vi "_FPGA_Const_RF_generator.vi"(6 "Enable":bool=TRUE, 7 "Reset_latch":bool, 9 "Amplitude_in(0-32768)":u16, 10 "Decycle_in":u32, 11 "Ticks_in":u32=10) -> (0 "Clk_out":bool, 2 "RF_out":fxp<+/-,16,14>)   [LabVIEW 2018]
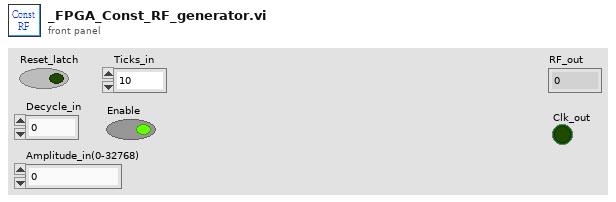
[diagram p1: front panel]
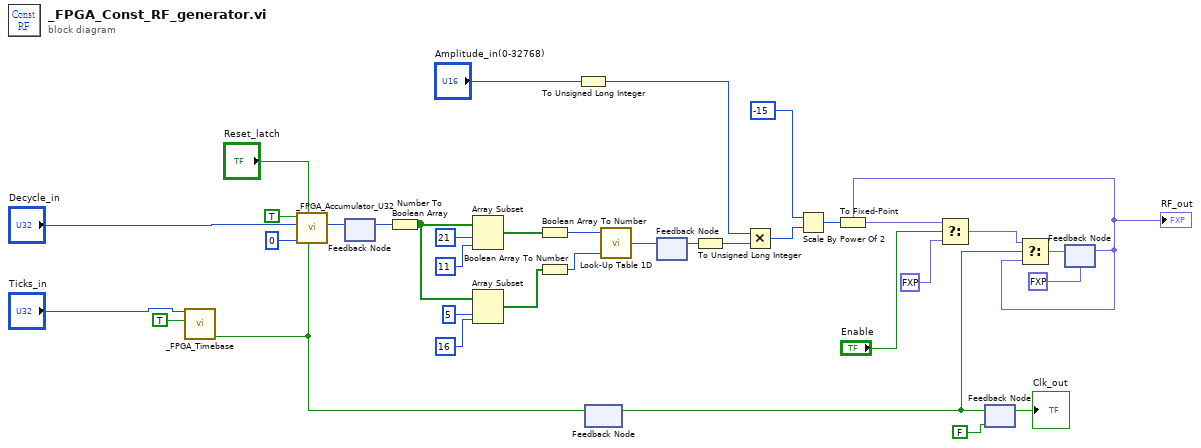
[diagram p0: block diagram]
diagram:
  n1 = call "_FPGA_Timebase.vi"("Enable"=TRUE, "Ticks"="Ticks_in") -> ("Clk_out"=w24:bool)  [unwired: 9 in]
  n2 = call "_FPGA_Accumulator_U32.vi"("Clk_in"=w24, "Reset_latch"="Reset_latch", "U32_shift_in"=u32 0, "U32_in"="Decycle_in", "Decrease / increase"=TRUE) -> ("Accumulated_U32_out"=w22:u32)  [unwired: 6 in]
  n3 = feedback #1() -> (w21:u32)  [unwired: 1 in]
  n4 = feedback-in #1(w22) -> ()
  n5 = Number To Boolean Array(number=w21) -> (Boolean array=w14:bool[])
  n6 = Array Subset(array=w14, index=21, length=11) -> (w18:bool[])
  n7 = Array Subset(array=w14, index=5, length=16) -> (w13:bool[])
  n8 = Boolean Array To Number(Boolean array=w18) -> (number=w17:u16)
  n9 = Boolean Array To Number(Boolean array=w13) -> (number=w12:u16)
  n10 = To Unsigned Long Integer(number="Amplitude_in(0-32768)") -> (unsigned 32bit integer=w7:u32)
  n11 = feedback #2() -> (w23:bool)  [unwired: 1 in]
  n12 = feedback-in #2(w24) -> ()
  n13 = call "Look-Up Table 1D"("address"=w17, "fractional index (x 2^16)"=w12) -> ("data out"=w9:u16)  [unwired: 7 in]
  n14 = feedback-in #3(w9) -> ()
  n15 = feedback #3() -> (w2:u16)  [unwired: 1 in]
  n16 = To Unsigned Long Integer(number=w2) -> (unsigned 32bit integer=w6:u32)
  n17 = Multiply(x=w7, y=w6) -> (x*y=w5:u32)
  n18 = Scale By Power Of 2(n=i16 -15, x=w5) -> (x*2^n=w3:u32)
  n19 = feedback #4(FALSE ("Clk_out")) -> (→"Clk_out":bool)
  n20 = feedback-in #4(w23) -> ()
  n21 = feedback #5(fxp<+/-,16,14> 0.0 ("sine")) -> (w11:fxp<+/-,17,15>)
  "RF_out" <- w11
  n22 = To Fixed-Point(fixed-point type=w11, number=w3) -> (fixed-point=w10:fxp<+/-,17,15>)
  n23 = Select(t=w10, s="Enable", f=fxp<+/-,17,15> 0.0) -> (s? t:f=w26:fxp<+/-,17,15>)
  n24 = Select(t=w26, s=w23, f=w11) -> (s? t:f=w31:fxp<+/-,17,15>)
  n25 = feedback-in #5(w31) -> ()
